vi "GetChannelName.vi"(8 "error in (no error)":errorcluster, 11 "ClassIn":refnum<class "Keysight335XX.lvclass">) -> (0 "error out":errorcluster, 3 "ClassOut":refnum<class "Keysight335XX.lvclass">)   [LabVIEW 2014, in "FGenPlugins.lvlib" / "Keysight335XX.lvclass"]
uses:
  Keysight335XX.lvclass
  MyPluginBaseClass/TypeDef/ChannelParamElement.ctl
  <vilib>/Utility/error.llb/Error Cluster From Error Code.vi
  <vilib>/ErrorRing/Error Ring.xnode
  MyPluginBaseClass/NISTFGenPluginsBase.lvclass
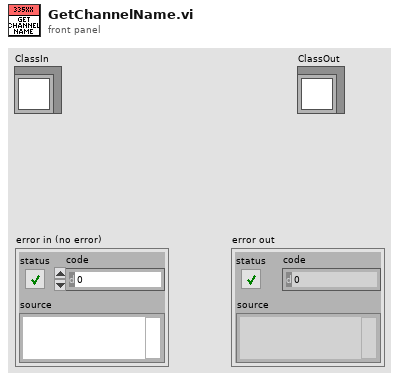
[diagram p1: front panel]
types:
  T1 = typedef "FGenPlugins.lvlib/NISTFGenPluginsBase.lvclass/ChannelParamElement.ctl" = cluster{"sName":string, "eOperateMode":u16, "bEnabled":bool, "eOutputMode":u16, "iIndex":i32, "iNameBufferSize":i32, "fGain":dbl}
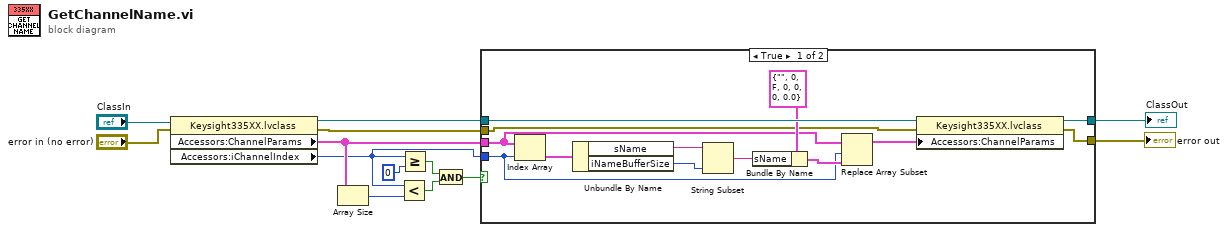
[diagram p0: block diagram]
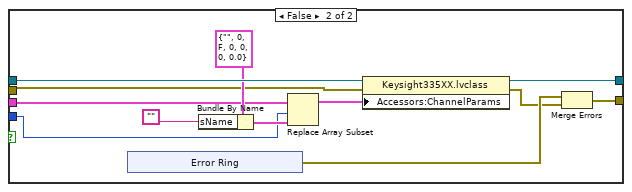
[diagram p2: hidden frame]
diagram:
  n1 = property class="Keysight335XX.lvclass"(reference="ClassIn", error in="error in (no error)") -> (reference out=w5:refnum<class "Keysight335XX.lvclass">, error out=w3:errorcluster, "Accessors:ChannelParams"=w10:T1[], "Accessors:iChannelIndex"=w1:i32)
  n2 = Array Size(array=w10) -> (size(s)=w9:i32)
  n3 = Less?(x=w1, y=w9) -> (x < y?=w8:bool)
  n4 = Greater Or Equal?(x=w1, y=0 ("x")) -> (x >= y?=w11:bool)
  n5 = And(x=w11, y=w8) -> (x .and. y?=w7:bool)
  n6 = case shown="True" w7 {
    tunnel: w10 -> [w19 w35]
    tunnel: w5 -> [w23 w38]
    tunnel: [w17 w33] -> w4
    tunnel: w3 -> [w16 w32]
    tunnel: [w15 w27] -> w2
    tunnel: w1 -> [w14 w30]
    frame True {
      n7 = Index Array(array=w19, index=w14) -> (element=w26:T1)
      n8 = Unbundle By Name(w26) -> ("sName"=w25:string, "iNameBufferSize"=w24:i32)
      n9 = String Subset(string=w25, length (rest)=w24) -> (substring=w22:string)  [unwired: 1 in]
      n10 = Bundle By Name(cluster=T1 {"sName"="", "eOperateMode"=0, "bEnabled"=FALSE, "eOutputMode"=0, "iIndex"=0, "iNameBufferSize"=0, "fGain"=0.0} ("ChannelParamElement"), "sName"=w22) -> (w20:T1)
      n11 = Replace Array Subset(array=w19, new element=w20, index=w14) -> (w18:T1[])
      n12 = property class="Keysight335XX.lvclass"(reference=w23, error in=w16, "Accessors:ChannelParams"=w18) -> (reference out=w17:refnum<class "Keysight335XX.lvclass">, error out=w15:errorcluster)
    }
    frame False {
      n13 = xnode "Error Ring"() -> ("error out"=w29:errorcluster)
      n14 = Bundle By Name(cluster=T1 {"sName"="", "eOperateMode"=0, "bEnabled"=FALSE, "eOutputMode"=0, "iIndex"=0, "iNameBufferSize"=0, "fGain"=0.0} ("ChannelParamElement"), "sName"="") -> (w36:T1)
      n15 = Replace Array Subset(array=w35, new element=w36, index=w30) -> (w34:T1[])
      n16 = property class="Keysight335XX.lvclass"(reference=w38, error in=w32, "Accessors:ChannelParams"=w34) -> (reference out=w33:refnum<class "Keysight335XX.lvclass">, error out=w28:errorcluster)
      n17 = Merge Errors(w29, w28) -> (w27:errorcluster)
    }
  }
  "error out" <- w2
  "ClassOut" <- w4
